vi "AUTOFLIM_Align_v2.vi"(0 "Z Scan Range":dbl, 2 "System no.":i32, 5 "Scan Termination":T1(ring), 11 "error in (no error)":errorcluster) -> (3 "Mesh out":dbl, 4 "Numeric 2":dbl, 6 "Numeric":dbl, 8 "Alignment Graph":dbl[][](array[numeric]), 14 "Z coordinate":dbl, 15 "error out":errorcluster)   [LabVIEW 2023]
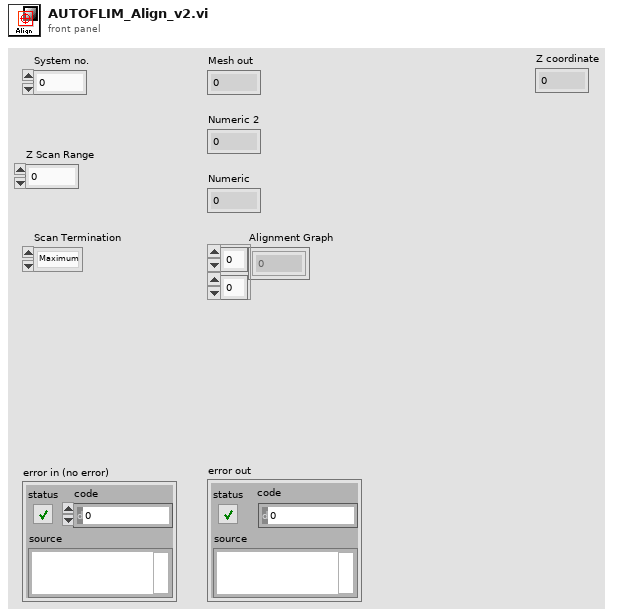
[diagram p1: front panel]
types:
  T1 = enum16{"Maximum", "End Position", "Center of scan"}
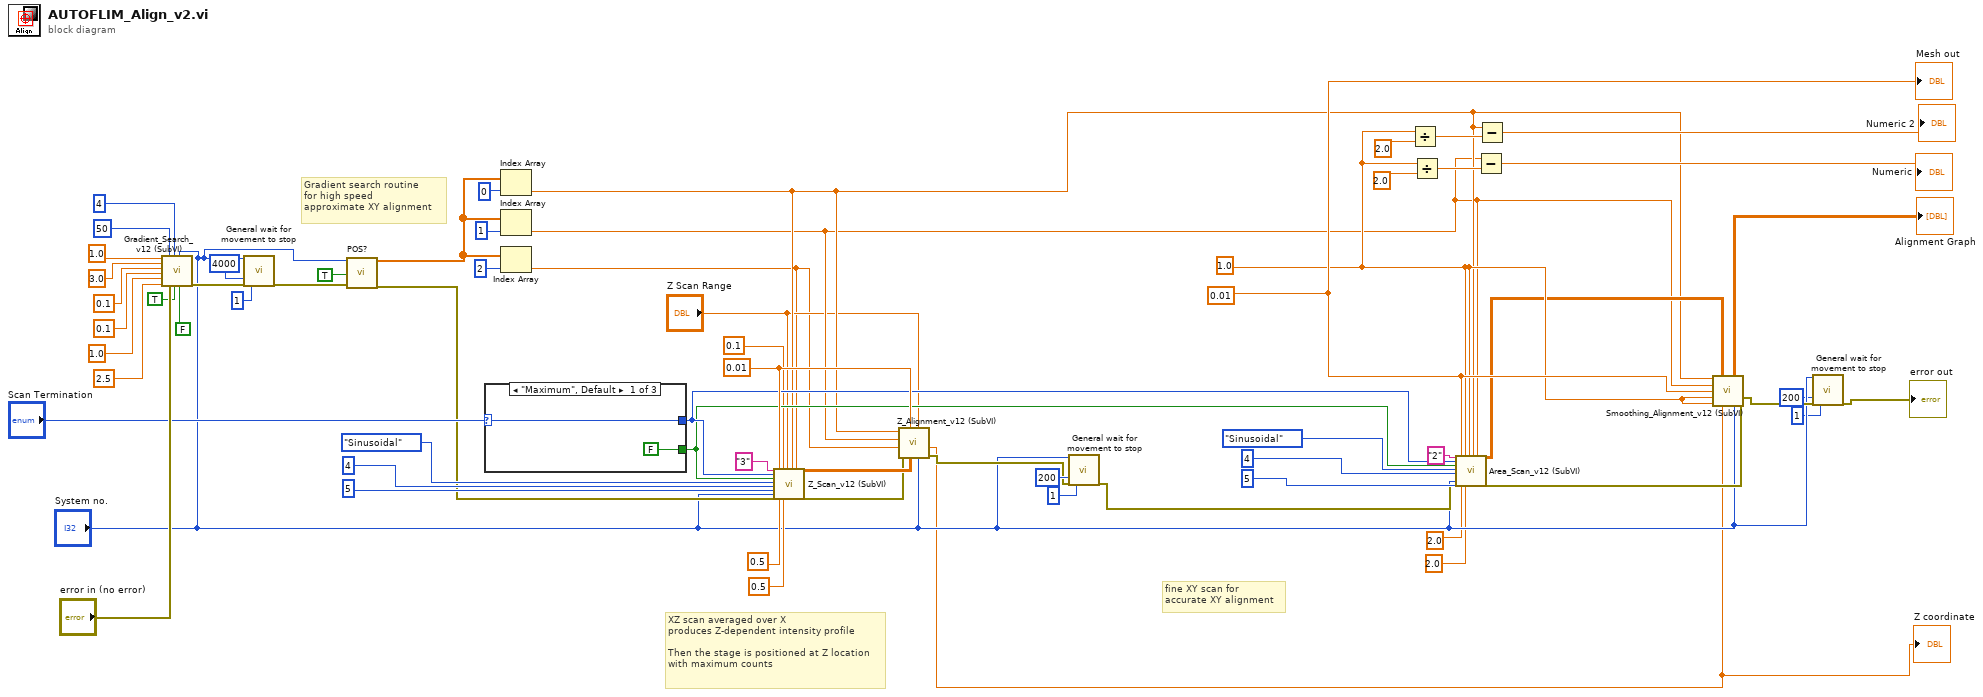
[diagram p0: block diagram]
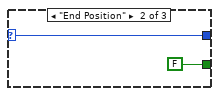
[diagram p2: hidden frame]
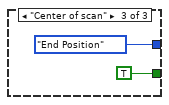
[diagram p3: hidden frame]
diagram:
  w65 = 0.01 ("Mesh in")
  w64 = 1.0 ("X Scan Range")
  w63 = 0.01 ("Z Mesh")
  # "fine XY scan for\naccurate XY alignment"
  # "XZ scan averaged over X\nproduces Z-dependent intensity profile\n\nThen the stage is positioned at Z location\nwith maximum counts"
  # "Gradient search routine\nfor high speed\napproximate XY alignment"
  n1 = call "Gradient_Search_v12 (SubVI).vi"("Speed factor"=1.0, "Max velocity"=3.0, "ML"=0.1, "Min Radius"=0.1, "Max Radius"=1.0, "GS Frequency"=2.5, "Max. dir. changes"=50, "error in (no error)"="error in (no error)", "Analog Input"=4, "Run?"=TRUE, "System no."="System no.", "Tracking"=FALSE) -> ("error out"=w33:errorcluster)  [unwired: 7 in]
  n2 = call "General wait for movement to stop.vi"("System no."="System no.", "Additional wait time, ms"=4000, "error in"=w33, "Polling cycle \ntime, ms"=1) -> ("error out"=w25:errorcluster)  [unwired: 4 in, 11 out]
  n3 = call "POS?.vi"("System no."="System no.", "All axes?"=TRUE, "error in"=w25) -> ("Position"=w20:dbl[], "error out"=w23:errorcluster)  [unwired: 2 in, 13 out]
  n4 = case shown="\"Maximum\", Default" "Scan Termination" {
    selector: "Scan Termination" -> [w67 w69 _]
    tunnel: [w67 w69 T1."End Position" ("Scan Termination")] -> w57
    tunnel: [FALSE FALSE TRUE] -> w56
    frame "Maximum", Default {
    }
    frame "End Position" {
    }
    frame "Center of scan" {
    }
  }
  n5 = Index Array(array=w20, index=0) -> (element=w18:dbl)
  n6 = Index Array(array=w20, index=1) -> (element=w17:dbl)
  n7 = Index Array(array=w20, index=2) -> (element=w4:dbl)
  n8 = call "Z_Scan_v12 (SubVI).vi"("Scan Axis"="3", "Scan Termination"=w57, "Center of Scan"=w56, "Scan Type"=enum16{"Sinusoidal", "Spiral"}."Sinusoidal", "Analog Input"=4, "Table rate"=5, "System no."="System no.", "error in (no error)"=w23, "Z Mesh"=w63, "Z-frequency"=0.5, "X Scan Range"=0.1, "Z-velocity"=0.5, "Z Scan Range"="Z Scan Range", "X Scan Center"=w18, "Z Scan Center"=w4) -> ("Intensity Graph"=w28:dbl[][], "error out"=w27:errorcluster)  [unwired: 8 in, 3 out]
  n9 = call "Z_Alignment_v12 (SubVI).vi"("System no."="System no.", "Z range"="Z Scan Range", "Intensity Graph"=w28, "Z Mesh"=w63, "error in (no error)"=w27, "Z"=w4, "Y"=w17, "X"=w18) -> ("error out"=w13:errorcluster, "Zout"=w5:dbl)  [unwired: 2 in]
  "Z coordinate" <- w5
  n10 = call "General wait for movement to stop.vi"("System no."="System no.", "Additional wait time, ms"=u32 200, "error in"=w13, "Polling cycle \ntime, ms"=u32 1 ("Polling cycle \ntime, ms")) -> ("error out"=w12:errorcluster)  [unwired: 4 in, 11 out]
  n11 = Divide(x=w64, y=2.0) -> (x/y=w39:dbl)
  n12 = Divide(x=w64, y=2.0) -> (x/y=w40:dbl)
  n13 = call "Area_Scan_v12 (SubVI).vi"("Step Axis"="2", "Scan Termination"=w57, "Center of Scan"=w56, "Scan Type"=enum16{"Sinusoidal", "Spiral"}."Sinusoidal", "Analog Input"=4, "Table rate"=5, "System no."="System no.", "error in (no error)"=w12, "Mesh in"=w65, "X-frequency"=2.0, "X Scan Range"=w64, "Y-velocity"=2.0 ("X-frequency"), "Y Scan Range"=w64, "X Scan Center"=w18, "Y Scan Center"=w17) -> ("Intensity Graph"=w29:dbl[][], "error out"=w26:errorcluster)  [unwired: 8 in, 3 out]
  n14 = Subtract(x=w17, y=w40) -> (x-y=→"Numeric":dbl)
  n15 = Subtract(x=w18, y=w39) -> (x-y=→"Numeric 2":dbl)
  n16 = call "Smoothing_Alignment_v12 (SubVI).vi"("X center"=w18, "Intensity Graph"=w29, "Y center"=w17, "Mesh"=w65, "X Scan Range"=w64, "Y Scan Range"=w64, "Z"=w5, "System no."="System no.", "error in (no error)"=w26) -> ("Alignment Graph"=→"Alignment Graph":dbl[][], "error out"=w11:errorcluster)  [unwired: 5 in]
  n17 = call "General wait for movement to stop.vi"("System no."="System no.", "Additional wait time, ms"=u32 200, "error in"=w11, "Polling cycle \ntime, ms"=u32 1 ("Polling cycle \ntime, ms")) -> ("error out"=→"error out":errorcluster)  [unwired: 4 in, 11 out]
  "Mesh out" <- w65
